vi "onCreated.vi"(8 "error in (no error)":errorcluster, 11 "XYStage":refnum<class "XYStage.lvclass">) -> (0 "error out":errorcluster, 3 "XYStage out":refnum<class "XYStage.lvclass">)   [LabVIEW 2013, in "XYStage.lvclass"]
doc: "JKI State Machine Objects (SMO) 1.0.4.18\nJKI - JKI\nCopyright (c) 2016, JKI"
uses:
  XYStage.lvclass
  <vilib>/JKI/JKI SMO/SMO/SMO.lvclass
  <vilib>/JKI/JKI SMO/SMO.Dictionary.Variant/SMO.Dictionary.Variant.lvclass
panel:
  # "For instructions on how to use the JKI State Machine Objects, examples and video tutorials, visit:\nhttp://jki.net/state-machine-objects/\n\nJKI State Machine Objects™\nhttp://jki.net/state-machine-objects/\nCopyright (C) 2005-2015, JKI <info@jki.net>\nALL RIGHTS RESERVED"
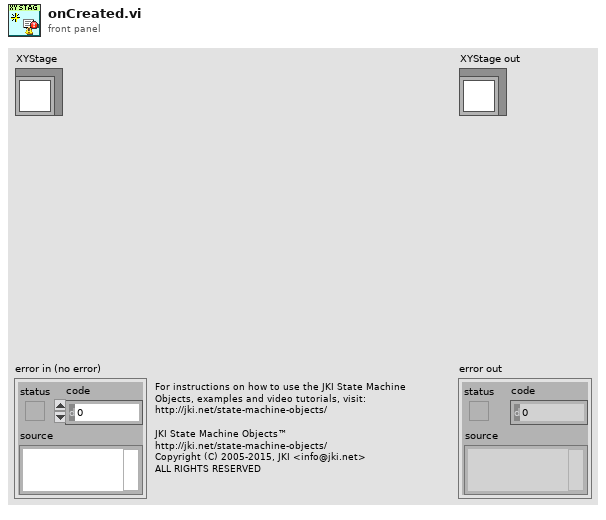
[diagram p1: front panel]
types:
  T1 = typedef "XYStage.lvclass/Dependencies--Cluster.ctl" = cluster{"Positions":refnum<class "SMO.Dictionary.Variant.lvclass">}
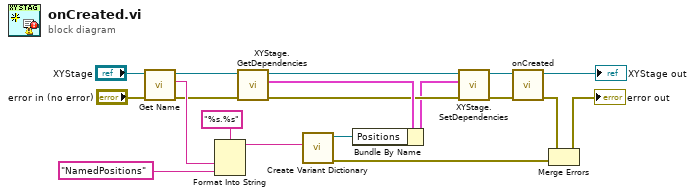
[diagram p0: block diagram]
diagram:
  n1 = call <vilib>:"Get Name.vi"("error in (no error)"="error in (no error)", "SMO"="XYStage") -> ("error out"=w11:errorcluster, "Name"=w16:string, "SMO out"=w12:refnum<class "XYStage.lvclass">)  [unwired: 7 in]
  n2 = Format Into String(format string="%s.%s", w16, "NamedPositions" ("format string")) -> (resulting string=w15:string)  [unwired: 2 in, 1 out]
  n3 = call "XYStage.GetDependencies.vi"("error in (no error)"=w11, "XYStage"=w12) -> ("error out"=w8:errorcluster, "Dependencies"=w13:T1, "XYStage out"=w10:refnum<class "XYStage.lvclass">)  [unwired: 7 in]
  n4 = call <vilib>:"Create Variant Dictionary.vi"("Subsystem Name (optional)"=w15) -> ("error out"=w5:errorcluster, "SMO.Dictionary.Variant out"=w14:refnum<class "SMO.Dictionary.Variant.lvclass">)  [unwired: 8 in, 1 out]
  n5 = Bundle By Name(cluster=w13, "Positions"=w14) -> (w6:T1)
  n6 = call "XYStage.SetDependencies.vi"("error in (no error)"=w8, "Dependencies"=w6, "XYStage"=w10) -> ("error out"=w7:errorcluster, "XYStage out"=w9:refnum<class "XYStage.lvclass">)  [unwired: 7 in]
  n7 = call-parent "onCreated.vi"("error in (no error)"=w7, "SMO"=w9) -> ("error out"=w4:errorcluster, "SMO out"=→"XYStage out":refnum<class "XYStage.lvclass">)  [unwired: 8 in]
  n8 = Merge Errors(w4, w5) -> (→"error out":errorcluster)
